vi "Get This VI.vi"(11 "Hello World Event in":refnum<class "Hello World Event.lvclass">) -> (2 "This VI":refnum<vi>)   [LabVIEW 2021, in "Hello World Event.lvlib" / "Hello World Event.lvclass"]
uses:
  Hello World Event.lvclass
  Hello World Event.lvclass/Hello World Event.ctl
  <vilib>/Nathan Davis/jettl/jettl/Event/Event.lvclass
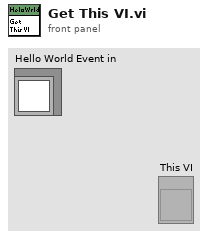
[diagram p1: front panel]
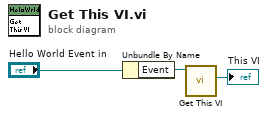
[diagram p0: block diagram]
diagram:
  n1 = Unbundle By Name("Hello World Event in") -> ("Event"=w2:refnum<class "Event.lvclass">)
  n2 = call-dynamic "Get This VI.vi"("jettl in"=w2) -> ("This VI"=→"This VI":refnum<vi>)  [unwired: 10 in]
